vi "Run_All_Tests.vi"() -> ()   [LabVIEW 2019]
panel:
  out "PhotonPoseEst":bool
  out "Packet":bool
  out "PhotonCamera":bool
  out "All Tests Finished":bool
  out "PhotonVisionUtil":bool
  # "FORMAL PHOTON VISION LIB LIBRARY TEST PROCEDURE"
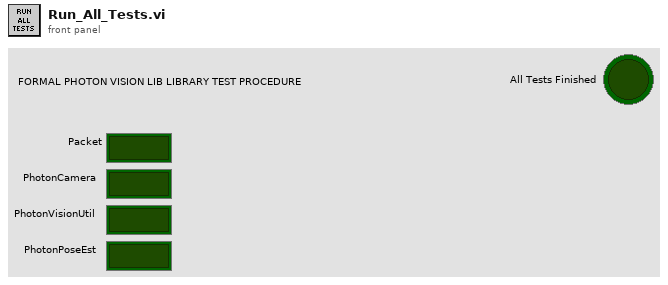
[diagram p1: front panel]
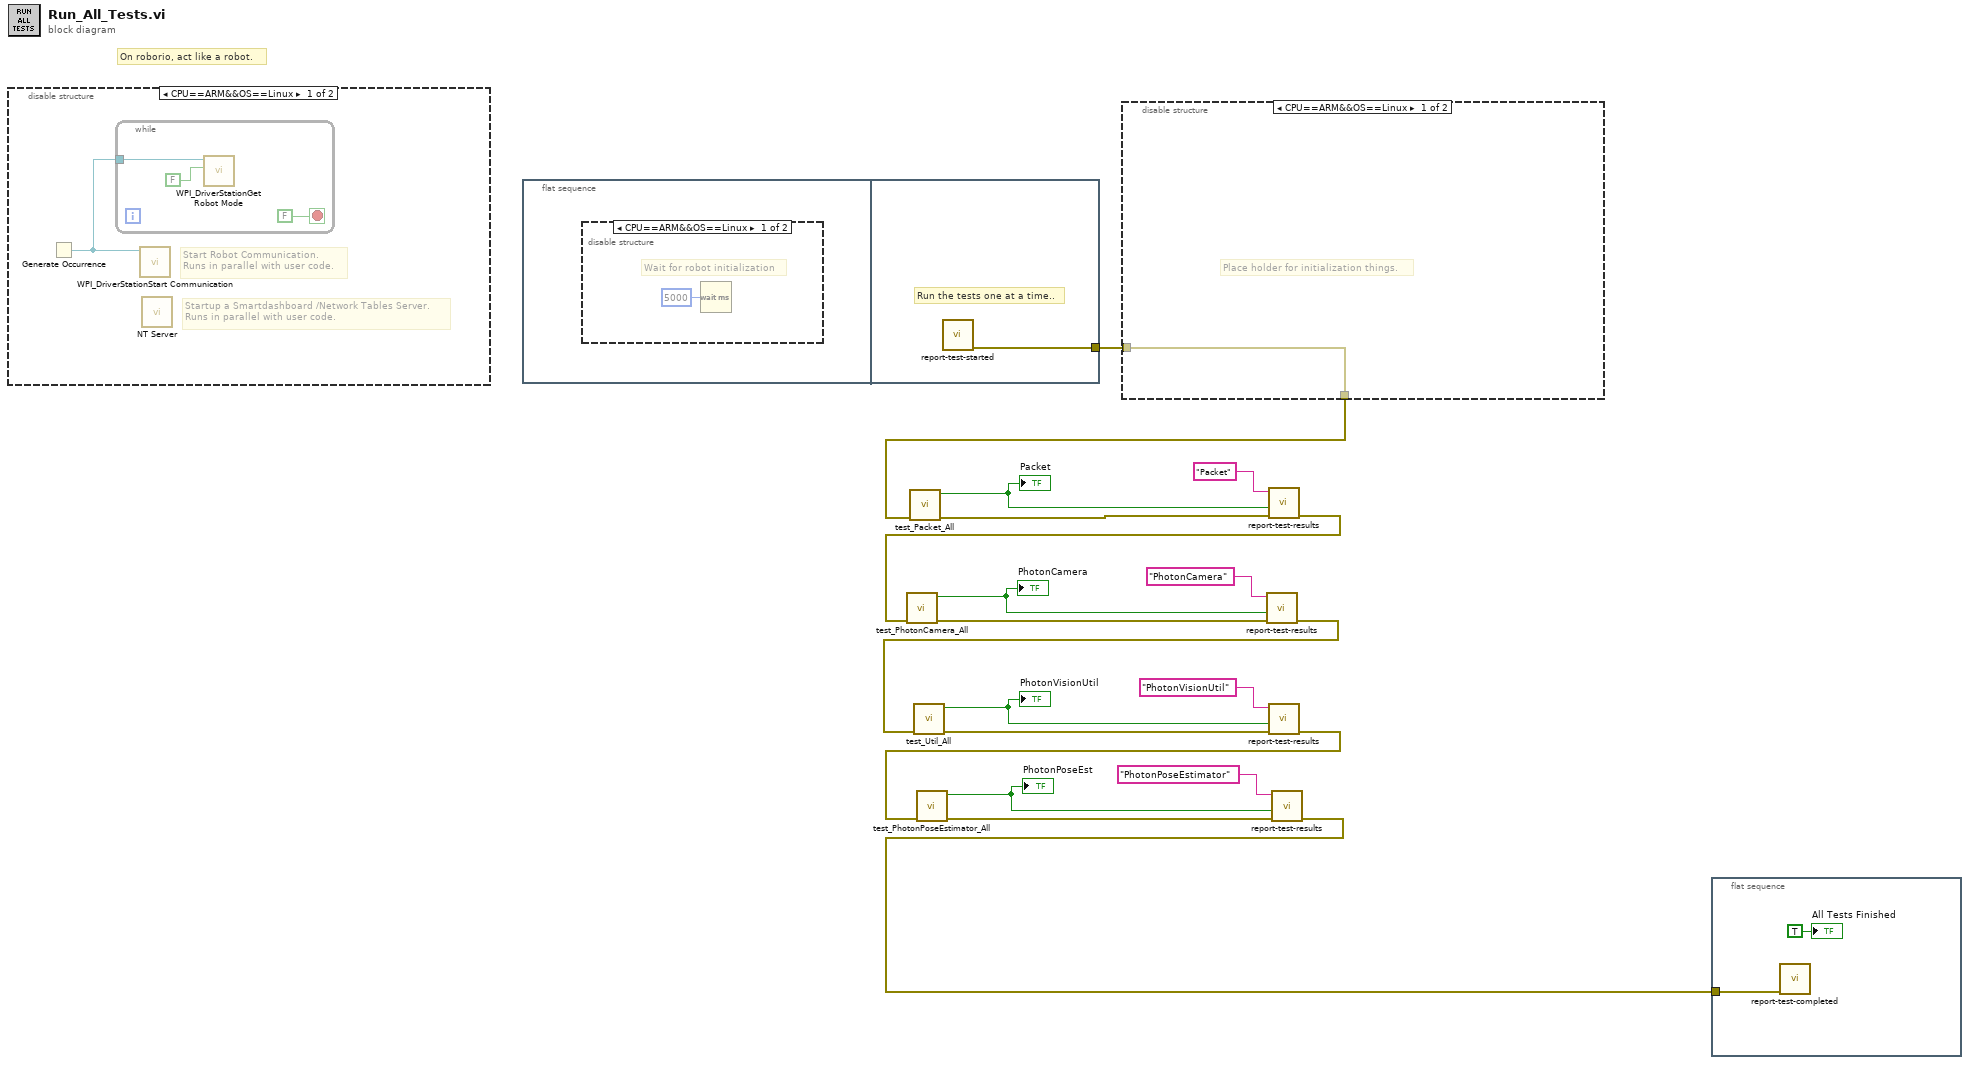
[diagram p0: block diagram]
diagram:
  # "On roborio, act like a robot."
  n1 = disable-structure shown="CPU==ARM&&OS==Linux" {
    frame condition #0 {
      # "Startup a Smartdashboard /Network Tables Server.\nRuns in parallel with user code."
      # "Start Robot Communication.\nRuns in parallel with user code."
      n2 = Generate Occurrence() -> (w19:refnum<k4>)
      n3 = while {
        tunnel: w19 -> [w22]
        stop <- FALSE stop-if-true
        n4 = call <vilib>:"WPI_DriverStationGet Robot Mode.vi"("Finish"=FALSE, "DS Occurrence"=w22) -> ()  [unwired: 10 out]
      }
      n5 = call <vilib>:"WPI_DriverStationStart Communication.vi"("occurrence"=w19) -> ()  [unwired: 2 in, 9 out]
      n6 = call <vilib>:"NT Server.vi"() -> ()  [unwired: 11 in, 1 out]
    }
    frame condition #1 (active) {
    }
  }
  n7 = flat-sequence {
    tunnel: [w24] -> w17
    frame #0 {
      n8 = disable-structure shown="CPU==ARM&&OS==Linux" {
        frame condition #0 {
          # "Wait for robot initialization"
          n9 = Wait (ms)(milliseconds to wait=u32 5000) -> ()  [unwired: 1 out]
        }
        frame condition #1 (active) {
        }
      }
    }
    frame #1 {
      # "Run the tests one at a time.."
      n10 = call "report-test-started.vi"() -> ("error out"=w24:errorcluster)  [unwired: 11 in]
    }
  }
  n11 = disable-structure shown="CPU==ARM&&OS==Linux" {
    disable-tunnel: w17 -> [w25 w26]
    disable-tunnel: [w25 w26] -> w7
    frame condition #0 {
      # "Place holder for initialization things."
    }
    frame condition #1 (active) {
    }
  }
  n12 = call "test_Packet_All.vi"("error in (no error)"=w7) -> ("error out"=w9:errorcluster, "Test Passed"=w8:bool)  [unwired: 9 in]
  "Packet" <- w8
  n13 = call "report-test-results.vi"("error in (no error)"=w9, "TestPassed"=w8, "Test Name"="Packet") -> ("error out"=w6:errorcluster)  [unwired: 8 in]
  n14 = call "test_PhotonCamera_All.vi"("error in (no error)"=w6) -> ("error out"=w12:errorcluster, "Test Passed"=w11:bool)  [unwired: 9 in]
  "PhotonCamera" <- w11
  n15 = call "report-test-results.vi"("error in (no error)"=w12, "TestPassed"=w11, "Test Name"="PhotonCamera") -> ("error out"=w13:errorcluster)  [unwired: 8 in]
  n16 = call "test_Util_All.vi"("error in (no error)"=w13) -> ("error out"=w16:errorcluster, "Test Passed"=w15:bool)  [unwired: 9 in]
  "PhotonVisionUtil" <- w15
  n17 = call "report-test-results.vi"("error in (no error)"=w16, "TestPassed"=w15, "Test Name"="PhotonVisionUtil") -> ("error out"=w2:errorcluster)  [unwired: 8 in]
  n18 = call "test_PhotonPoseEstimator_All.vi"("error in (no error)"=w2) -> ("error out"=w4:errorcluster, "Test Passed"=w3:bool)  [unwired: 9 in]
  "PhotonPoseEst" <- w3
  n19 = call "report-test-results.vi"("error in (no error)"=w4, "TestPassed"=w3, "Test Name"="PhotonPoseEstimator") -> ("error out"=w1:errorcluster)  [unwired: 8 in]
  n20 = flat-sequence {
    tunnel: w1 -> [w27]
    frame #0 {
      n21 = call "report-test-completed.vi"("error in (no error)"=w27) -> ()  [unwired: 10 in, 1 out]
      "All Tests Finished" <- TRUE ("All Tests Finished")
    }
  }
